vi "Process Pulse.vi"(8 "error in (no error)":errorcluster, 10 "Input":T2={"From"="broadcaster", "To"="broadcaster", "Pulse"=FALSE}, 11 "Broadcaster in":refnum<class "Broadcaster.lvclass">) -> (0 "error out":errorcluster, 2 "Outputs":T1(array[cluster]), 3 "Broadcaster out":refnum<class "Broadcaster.lvclass">)   [LabVIEW 2021, in "Broadcaster.lvclass"]
uses:
  Broadcaster.lvclass
  Broadcaster.lvclass/Broadcaster.ctl
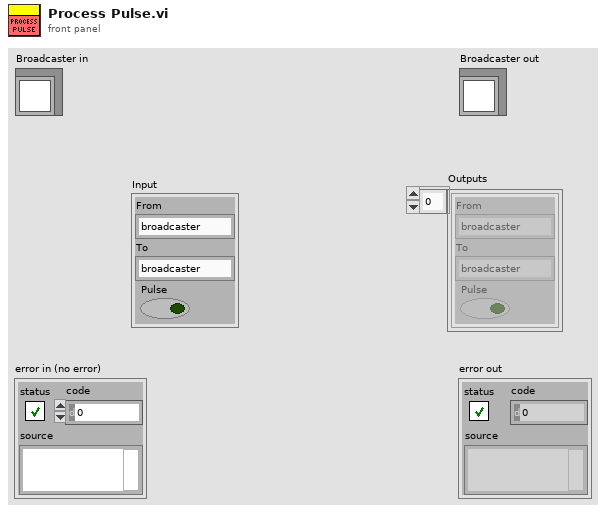
[diagram p1: front panel]
types:
  T1 = cluster{"From":string, "To":string, "Pulse":bool}[]
  T2 = cluster{"From":string, "To":string, "Pulse":bool}
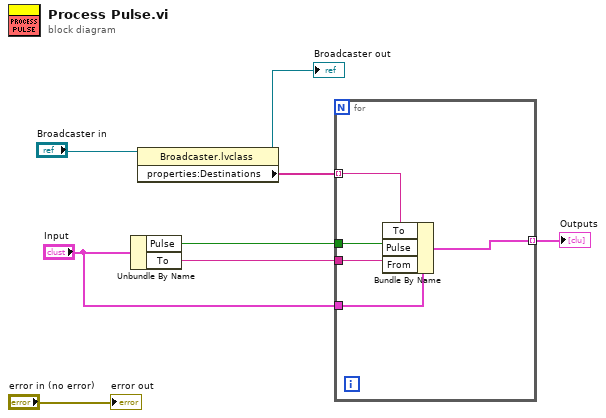
[diagram p0: block diagram]
diagram:
  n1 = Unbundle By Name("Input") -> ("Pulse"=w5:bool, "To"=w1:string)
  n2 = property class="Broadcaster.lvclass"(reference="Broadcaster in") -> (reference out=→"Broadcaster out":refnum<class "Broadcaster.lvclass">, "properties:Destinations"=w6:string[])  [unwired: 1 in, 1 out]
  n3 = for {
    tunnel: w6 -> [w12] mode=indexing
    tunnel: w5 -> [w13]
    tunnel: [w11] -> w4 mode=indexing
    tunnel: "Input" -> [w10]
    tunnel: w1 -> [w9]
    n4 = Bundle By Name(cluster=w10, "To"=w12, "Pulse"=w13, "From"=w9) -> (w11:T2)
  }
  "Outputs" <- w4
  "error out" <- "error in (no error)"
